vi "getControlData_distEst.vi"(11 "system matricec path":path=path "C:/Users/arnold/Documents/MATLAB/AFM_MPC/data/MPCControls01.csv") -> (1 "AllMatrix":dbl[](array[numeric]), 3 "ControlParams":T2={"umax"=3.0, "Ns_obs/cntrl"=0, "ref_f_VEC"=[0.0, 0.0], "du_max"=0.0, "Nbar"=0.0}, 4 "ControlMatrices":T1)   [LabVIEW 2017]
doc: "Reads the MPC controller data from a csv file. The format is specified as:\n\n[Ns, ref_f_x, ref_f_y, Nux, Nuy, umax, ]\nbeta, du_max, maxIter, Nmpc, Ns_mpc] \n[AllMatrix(:)' ]"
uses:
  fpga_VIs/fpga_subVIs_ssxy/fixed-point-ss/typeDefs/FXPControlParams_distEst.ctl
  ObserverMatrices.ctl
  <vilib>/Utility/file.llb/Read From Spreadsheet File (DBL).vi
panel:
  out "all rows":dbl[][](array[numeric]) format="%0.3f"
  out "subarray":dbl[](array[numeric])
  # "Reads the MPC controller data from a csv file. The format is specified as:\n\n[Ns, ref_f_x, ref_f_y, Nux, Nuy, umax, ]\nbeta, du_max, maxIter, Nmpc, Ns_mpc] \n[AllMatrix(:)'                                              ]"
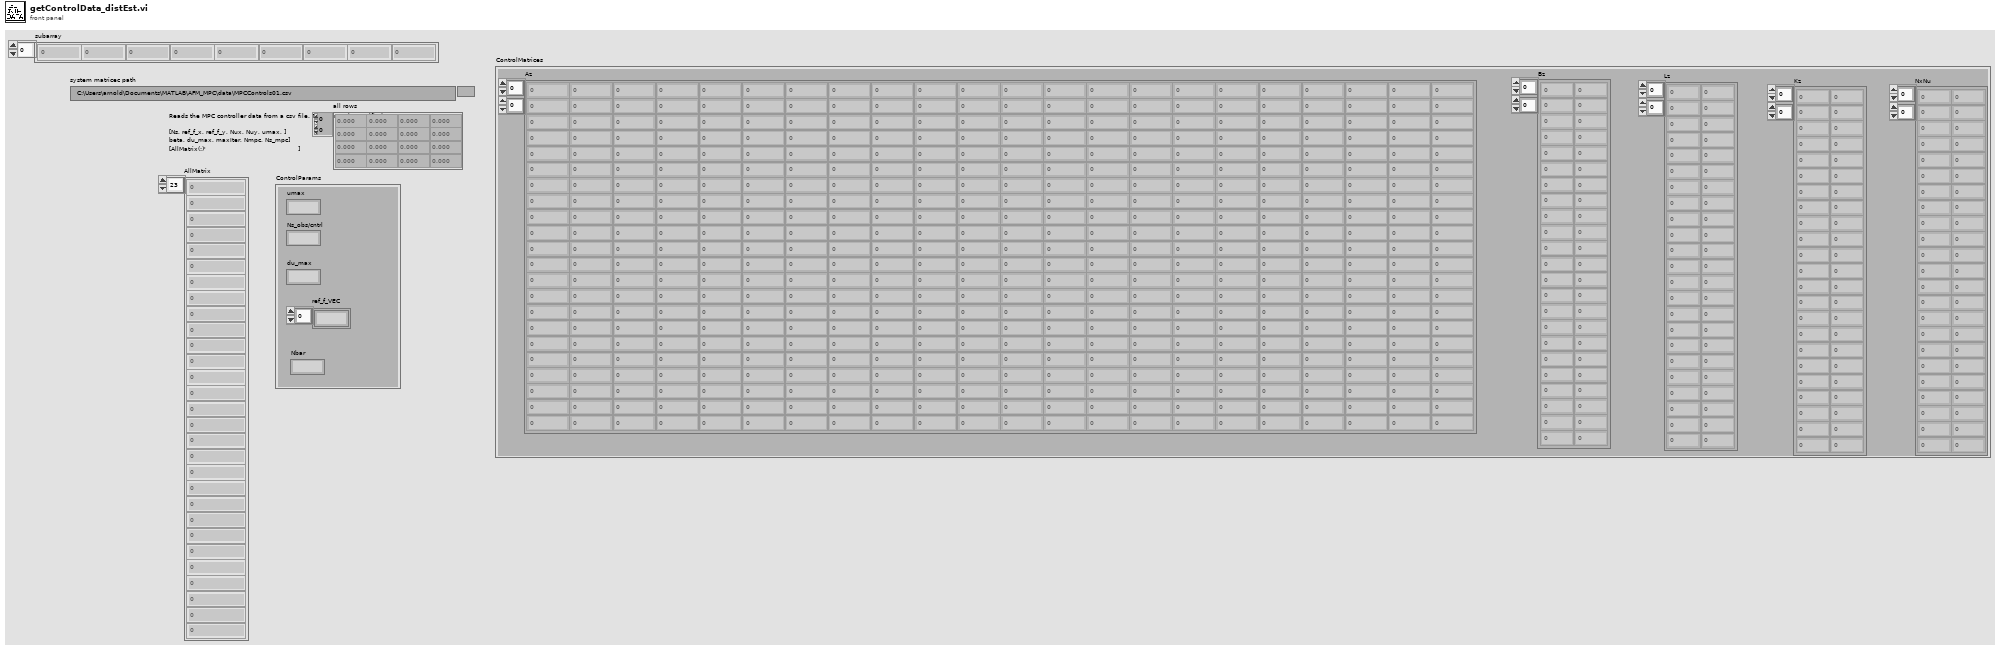
[diagram p1: front panel]
types:
  T1 = typedef "ObserverMatrices.ctl" = cluster{"Az":fxp<+/-,32,4>[][], "Bz":dbl[][], "Lz":dbl[][], "Kz":dbl[][], "NxNu":dbl[][]}
  T2 = typedef "FXPControlParams_distEst.ctl" = cluster{"umax":fxp<+/-,18,5>, "Ns_obs/cntrl":u8, "ref_f_VEC":fxp<+/-,32,5>[], "du_max":fxp<+/-,18,5>, "Nbar":fxp<+/-,32,5>}
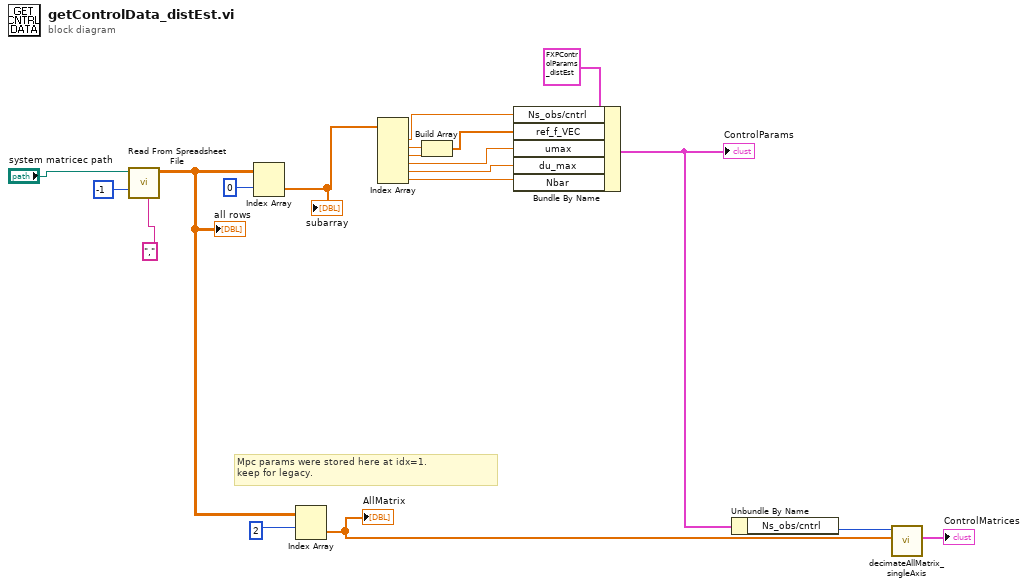
[diagram p0: block diagram]
diagram:
  # "Mpc params were stored here at idx=1.\nkeep for legacy."
  n1 = call-poly <vilib>:"Read From Spreadsheet File.vi"("delimiter (\\t)"=",", "number of rows (all:-1)"=-1, "file path (dialog if empty)"="system matricec path") -> ("all rows"=w10:dbl[][])  [unwired: 4 in, 4 out]
  "all rows" <- w10
  n2 = Index Array(array=w10, index (row)=0 ("dimension size")) -> (element=w11:dbl[])  [unwired: 1 in]
  "subarray" <- w11
  n3 = Index Array(array=w10, index (row)=2 ("dimension size")) -> (element=w1:dbl[])  [unwired: 1 in]
  "AllMatrix" <- w1
  n4 = Index Array(array=w11) -> (element #1=w13:dbl, element #2=w16:dbl, element #3=w15:dbl, element #4=w4:dbl, element #5=w3:dbl, element #6=w2:dbl)  [unwired: 6 in]
  n5 = Build Array(w16, w15) -> (w12:dbl[])
  n6 = Bundle By Name(cluster=T2 {"umax"=3.0, "Ns_obs/cntrl"=0, "ref_f_VEC"=[0.0, 0.0], "du_max"=0.0, "Nbar"=0.0} ("ControlParams 2"), "Ns_obs/cntrl"=w13, "ref_f_VEC"=w12, "umax"=w4, "du_max"=w3, "Nbar"=w2) -> (w7:T2)
  "ControlParams" <- w7
  n7 = Unbundle By Name(w7) -> ("Ns_obs/cntrl"=w5:u8)
  n8 = call "decimateAllMatrix_singleAxis.vi"("AllMatrix"=w1, "NS_obs/cntrl"=w5) -> ("ControlMatrices"=→"ControlMatrices":T1)  [unwired: 8 in, 1 out]
